vi "Verify Gen Cal.vi"(10 "input string":string) -> (0 "actual vrect":string, 1 "expected vrect":string, 2 "actual therm":string, 3 "expected therm":string, 5 "Validation Passed?":bool)   [LabVIEW 2010]
doc: "This function parses an xPG General Calibration Status string and compares the \"therm\" and \"vrect\" parameters."
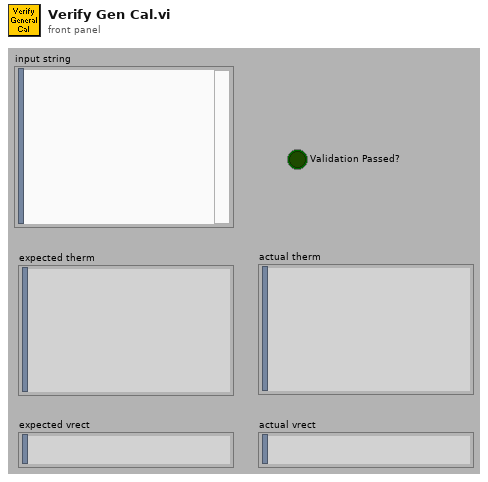
[diagram p1: front panel]
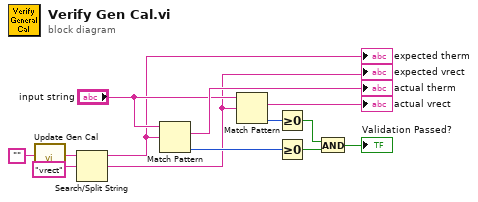
[diagram p0: block diagram]
diagram:
  n1 = call "Update Gen Cal.vi"("Input String"="") -> ("Output String"=w8:string)  [unwired: 10 in]
  n2 = Search/Split String(string=w8, search string/char (-)="vrect" ("regular expression")) -> (substring before match=w2:string, match + rest of string=w1:string)  [unwired: 1 in, 1 out]
  "expected therm" <- w2
  "expected vrect" <- w1
  n3 = Match Pattern(string="input string", regular expression=w2) -> (match substring=→"actual therm":string, offset past match=w13:i32)  [unwired: 1 in, 2 out]
  n4 = Match Pattern(string="input string", regular expression=w1) -> (match substring=→"actual vrect":string, offset past match=w12:i32)  [unwired: 1 in, 2 out]
  n5 = Greater Or Equal To 0?(x=w12) -> (x >= 0?=w10:bool)
  n6 = Greater Or Equal To 0?(x=w13) -> (x >= 0?=w11:bool)
  n7 = And(x=w10, y=w11) -> (x .and. y?=→"Validation Passed?":bool)
